vi "GetType.vi"(8 "error in (no error)":errorcluster, 11 "Write calibration curves to instruments Msg":refnum<class "Write calibration curves to instruments Msg.lvclass">) -> (0 "error out":errorcluster, 2 "Data Sample":variant, 3 "Write calibration curves to instruments Msg":refnum<class "Write calibration curves to instruments Msg.lvclass">)   [LabVIEW 2016, in "LS218.lvlib" / "Write calibration curves to instruments Msg.lvclass"]
uses:
  Write calibration curves to instruments Msg.lvclass
  Write calibration curves to instruments Msg.lvclass/Write calibration curves to instruments Msg.ctl
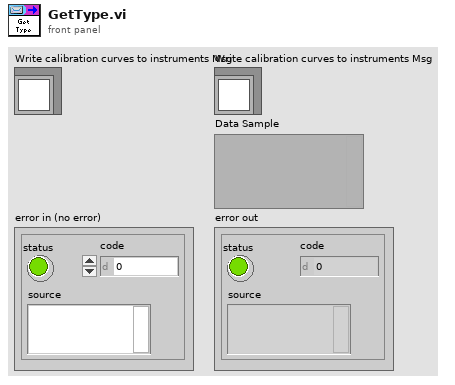
[diagram p1: front panel]
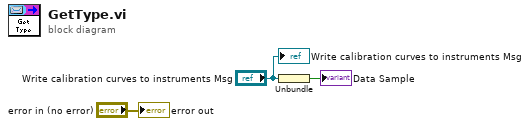
[diagram p0: block diagram]
diagram:
  n1 = Unbundle("Write calibration curves to instruments Msg") -> (→"Data Sample":bool)
  "error out" <- "error in (no error)"
  "Write calibration curves to instruments Msg" <- "Write calibration curves to instruments Msg"
